vi "Acquisition Message Loop.vi"(8 "error in (no error)":errorcluster, 9 "Data Queue":refnum<queue>, 10 "Data Notifier":refnum<notifier>, 11 "Message Queues":T1) -> (0 "error out":errorcluster)   [LabVIEW 2013, in "Acquisition.lvlib"]
doc: "Message loop for handling messages pertaining to the acquisition of data from the hardware."
uses:
  Acquisition.lvlib
  support/Message Queue/All Message Queues.ctl
  support/Message Queue/Message Cluster.ctl
  Hardware Configuration.ctl
  Acquisition State.ctl
  support/Message Queue/Enqueue Message (Single).vi
  <vilib>/Utility/error.llb/Error Cluster From Error Code.vi
  <vilib>/ErrorRing/Error Ring.xnode
  support/Message Queue/Message Queue.lvlib
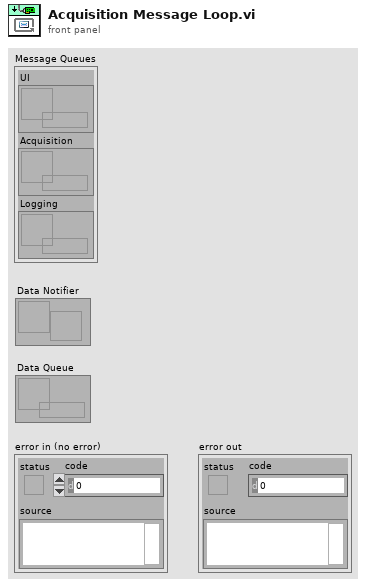
[diagram p1: front panel]
types:
  T1 = typedef "Message Queue.lvlib/All Message Queues.ctl" = cluster{"UI":refnum<queue>, "Acquisition":refnum<queue>, "Logging":refnum<queue>}
  T2 = typedef "Acquisition.lvlib/Hardware Configuration.ctl" = cluster{"DAQmx Channel":tag, "Max Input":dbl, "Min Input":dbl, "Sample Rate":dbl, "DAQmx Task":refnum<k21>}
  T3 = typedef "Acquisition.lvlib/Acquisition State.ctl" = enum16{"Idle", "Acquiring"}
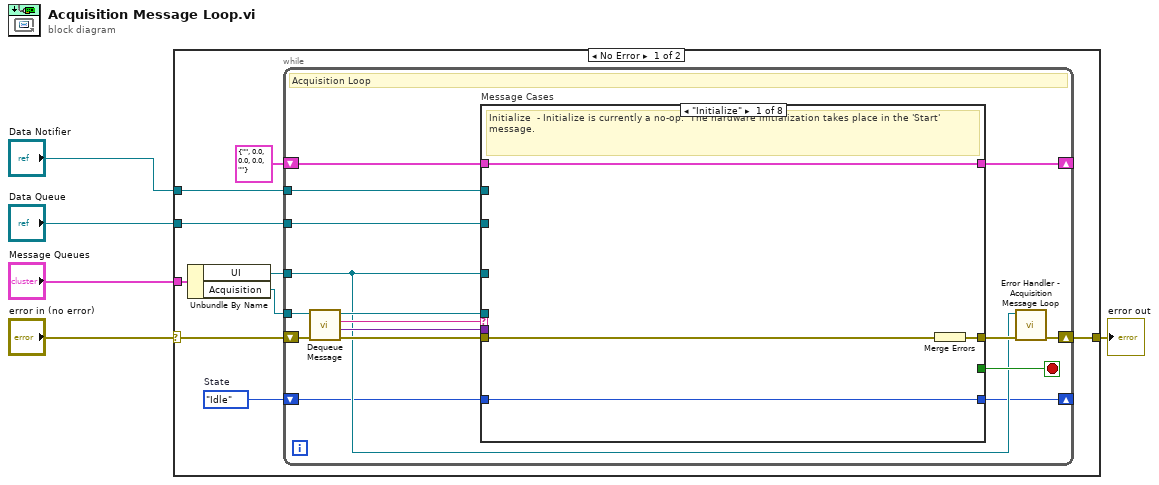
[diagram p0: block diagram]
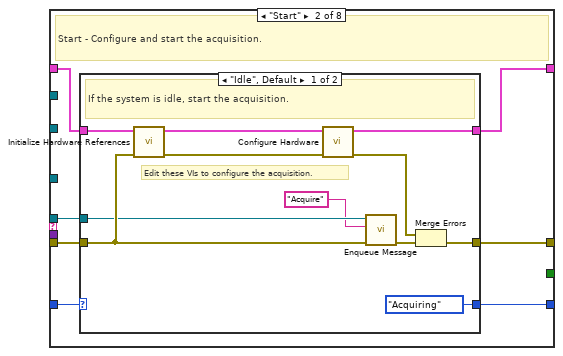
[diagram p2: hidden frame]
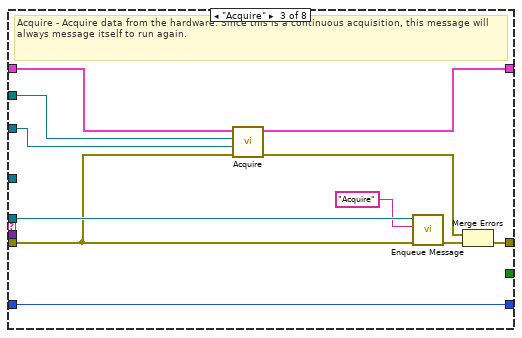
[diagram p4: hidden frame]
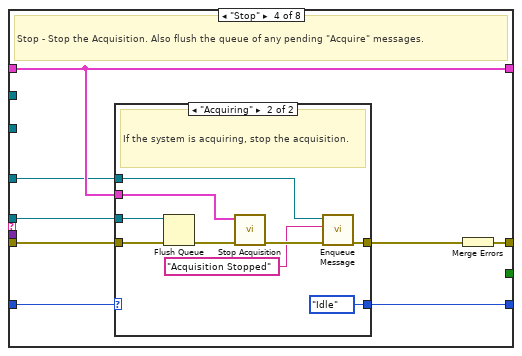
[diagram p5: hidden frame]
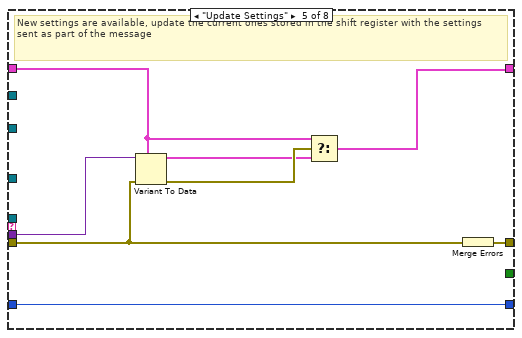
[diagram p7: hidden frame]
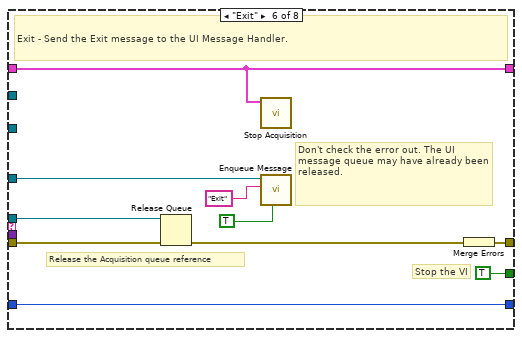
[diagram p8: hidden frame]
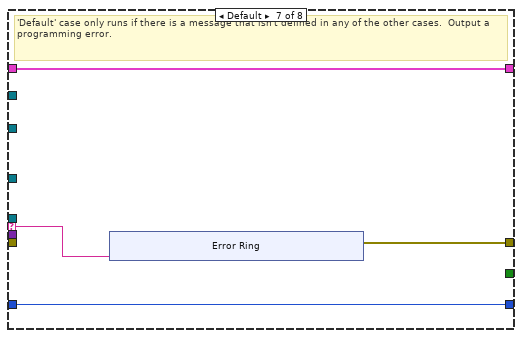
[diagram p9: hidden frame]
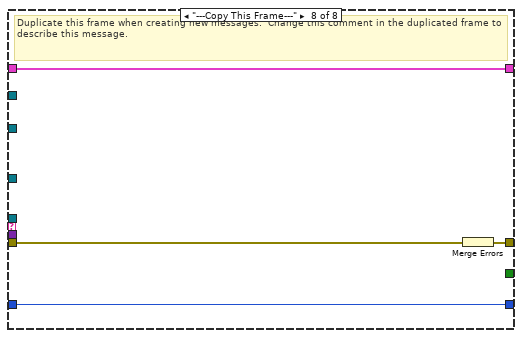
[diagram p10: hidden frame]
diagram:
  n1 = case shown="No Error" "error in (no error)" {
    selector: "error in (no error)" -> [w10 w119]
    tunnel: "Message Queues" -> [w14 _]
    tunnel: [w12 w119] -> w4
    tunnel: "Data Notifier" -> [w8 _]
    tunnel: "Data Queue" -> [w7 _]
    frame No Error {
      w6 = Acquisition_State."Idle"  # State
      n2 = Unbundle By Name(w14) -> ("UI"=w9:refnum<queue>, "Acquisition"=w13:refnum<queue>)
      n3 = while {
        tunnel: w13 -> [w22]
        shift-right: [w29] -> _
        shift-left: T2 {"DAQmx Channel"="", "Max Input"=0.0, "Min Input"=0.0, "Sample Rate"=0.0, "DAQmx Task"=""} ("Data Cluster") -> [w30]
        shift-right: [w18] -> w12
        shift-left: w10 -> [w27]
        tunnel: w9 -> [w17]
        tunnel: w8 -> [w21]
        tunnel: w7 -> [w20]
        shift-right: [w15] -> _
        shift-left: w6 -> [w16]
        stop <- w28 stop-if-true
        # "Acquisition Loop"
        n4 = call "Dequeue Message.vi"("error in (no error)"=w27, "Message Queue"=w22) -> ("error out"=w26:errorcluster, "Message Data"=w24:variant, "Message"=w25:string, "dup Message Queue"=w23:refnum<queue>)  [unwired: 6 in]
        n5 = case "Message Cases" shown="\"Initialize\"" w25 {
          selector: w25 -> [_ _ _ _ _ _ w106 _]
          tunnel: w23 -> [_ w38 w64 w71 _ w96 _ _]
          tunnel: w26 -> [w33 w39 w63 w73 w87 w100 _ w118]
          tunnel: [w34 w41 w66 w74 w93 w102 w105 w116] -> w19
          tunnel: w30 -> [w32 w40 w60 w72 w89 w95 w107 w117]
          tunnel: [w32 w37 w61 w72 w88 w95 w107 w117] -> w29
          tunnel: [_ _ _ _ _ TRUE _ _] -> w28
          tunnel: w24 -> [_ _ _ _ w92 _ _ _]
          tunnel: w17 -> [_ _ _ w70 _ w101 _ _]
          tunnel: w21 -> [_ _ w58 _ _ _ _ _]
          tunnel: w20 -> [_ _ w57 _ _ _ _ _]
          tunnel: w16 -> [w31 w36 w56 w69 w86 w94 w104 w115]
          tunnel: [w31 w35 w56 w68 w86 w94 w104 w115] -> w15
          frame "Initialize" {
            # "Initialize  - Initialize is currently a no-op.  The hardware initialization takes place in the 'Start' message."
            n6 = Merge Errors(w33) -> (w34:errorcluster)
          }
          frame "Start" {
            # "Start - Configure and start the acquisition."
            n7 = case shown="\"Idle\", Default" w36 {
              selector: w36 -> [_ w53]
              tunnel: [w52 w55] -> w41
              tunnel: w40 -> [w51 w54]
              tunnel: w39 -> [w50 w55]
              tunnel: w38 -> [w48 _]
              tunnel: [w44 w54] -> w37
              tunnel: [Acquisition_State."Acquiring" ("State") w53] -> w35
              frame "Idle", Default {
                # "Edit these VIs to configure the acquisition."
                # "If the system is idle, start the acquisition."
                n8 = call "Initialize Hardware References.vi"("error in (no error)"=w50, "Hardware Resources in"=w51) -> ("error out"=w47:errorcluster, "Hardware Resources out"=w45:T2)  [unwired: 8 in]
                n9 = call "Configure Hardware.vi"("error in (no error)"=w47, "Hardware Resources in"=w45) -> ("error out"=w46:errorcluster, "Hardware Resources out"=w44:T2)  [unwired: 8 in]
                n10 = call-poly "Enqueue Message.vi"("error in (no error)"=w50, "Message"="Acquire", "Message Queue"=w48) -> ("error out"=w49:errorcluster)  [unwired: 7 in, 1 out]
                n11 = Merge Errors(w46, w49) -> (w52:errorcluster)
              }
              frame "Acquiring" {
                # "The system is already acquiring. Ignore the \"Start\" message."
              }
            }
          }
          frame "Acquire" {
            # "Acquire - Acquire data from the hardware. Since this is a continuous acquisition, this message will always message itself to run again."
            n12 = call "Acquire.vi"("error in (no error)"=w63, "Data Queue"=w57, "Data Notifier"=w58, "Hardware Resources in"=w60) -> ("error out"=w62:errorcluster, "Hardware Resources out"=w61:T2)  [unwired: 6 in]
            n13 = call-poly "Enqueue Message.vi"("error in (no error)"=w63, "Message"="Acquire", "Message Queue"=w64) -> ("error out"=w65:errorcluster)  [unwired: 7 in, 1 out]
            n14 = Merge Errors(w62, w65) -> (w66:errorcluster)
          }
          frame "Stop" {
            # "Stop - Stop the Acquisition. Also flush the queue of any pending \"Acquire\" messages."
            n15 = case shown="\"Acquiring\"" w69 {
              selector: w69 -> [w76 _]
              tunnel: w73 -> [w75 w85]
              tunnel: w72 -> [_ w84]
              tunnel: w71 -> [_ w82]
              tunnel: w70 -> [_ w81]
              tunnel: [w76 Acquisition_State."Idle" ("State")] -> w68
              tunnel: [w75 w79] -> w67
              frame "Idle", Default {
                # "The system is already idle. Ignore the \"Stop\" message."
              }
              frame "Acquiring" {
                # "If the system is acquiring, stop the acquisition."
                n16 = Flush Queue(queue=w82, error in (no error)=w85) -> (error out=w83:errorcluster)  [unwired: 2 out]
                n17 = call "Stop Acquisition.vi"("error in (no error)"=w83, "Hardware Resources in"=w84) -> ("error out"=w80:errorcluster)  [unwired: 9 in]
                n18 = call-poly "Enqueue Message.vi"("error in (no error)"=w80, "Message"="Acquisition Stopped", "Message Queue"=w81) -> ("error out"=w79:errorcluster)  [unwired: 7 in, 1 out]
              }
            }
            n19 = Merge Errors(w67) -> (w74:errorcluster)
          }
          frame "Update Settings" {
            # "New settings are available, update the current ones stored in the shift register with the settings sent as part of the message"
            n20 = Variant To Data(error in=w87, type=w89, Variant=w92) -> (data=w90:T2, error out=w91:errorcluster)
            n21 = Select(t=w89, s=w91, f=w90) -> (s? t:f=w88:T2)
            n22 = Merge Errors(w87) -> (w93:errorcluster)
          }
          frame "Exit" {
            # "Don't check the error out. The UI message queue may have already been released."
            # "Release the Acquisition queue reference"
            # "Stop the VI"
            # "Exit - Send the Exit message to the UI Message Handler."
            n23 = Release Queue(queue=w96, error in (no error)=w100) -> (error out=w97:errorcluster)  [unwired: 1 in, 2 out]
            n24 = call "Stop Acquisition.vi"("Hardware Resources in"=w95) -> ()  [unwired: 10 in, 1 out]
            n25 = call-poly "Enqueue Message.vi"("Priority Message? (F)"=TRUE, "Message"="Exit", "Message Queue"=w101) -> ()  [unwired: 7 in, 2 out]
            n26 = Merge Errors(w97) -> (w102:errorcluster)
          }
          frame Default {
            # "'Default' case only runs if there is a message that isn't defined in any of the other cases.  Output a programming error."
            n27 = xnode "Error Ring"("parameter 0"=w106) -> ("error out"=w105:errorcluster)
          }
          frame "---Copy This Frame---" {
            # "Duplicate this frame when creating new messages.  Change this comment in the duplicated frame to describe this message."
            n28 = Merge Errors(w118) -> (w116:errorcluster)
          }
        }
        n29 = call "Error Handler - Acquisition Message Loop.vi"("error in (no error)"=w19, "Message Queue"=w17) -> ("dup error in"=w18:errorcluster)  [unwired: 8 in, 1 out]
      }
    }
    frame Error {
    }
  }
  "error out" <- w4
